vi "VI Server_Open VI Controls Refs_Labels_ApplicationRefInput.vi"(8 "error in (no error)":errorcluster, 10 "port number or service name (3363)":u16=3363, 11 "Target VI Path":path) -> (0 "error out":errorcluster, 3 "VI Server Cluster.OUT":T1)   [LabVIEW 2020, in "VI Server Toolkit LV2013.lvlib"]
doc: "Generates the VI Server Cluster with application input. Uses VI Server port to access application.\nThis VI used in compiled LabVIEW applications to access controls in LabVIEW development environment."
uses:
  VI Server Toolkit LV2013.lvlib
  VI Server_TypeDefs/VI Server_RefsCluster.ctl
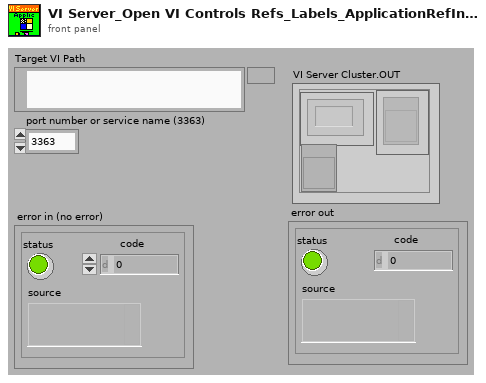
[diagram p1: front panel]
types:
  T1 = typedef "VI Server_RefsCluster.ctl" = cluster{"Labels":string[], "Refs":refnum<vi>[], "VI Ref":refnum<vi>}
  T2 = enum32{"invalid app kind", "Development System", "Run Time System", "Student Edition", "Embedded LabVIEW", "Evaluation", "Custom"}
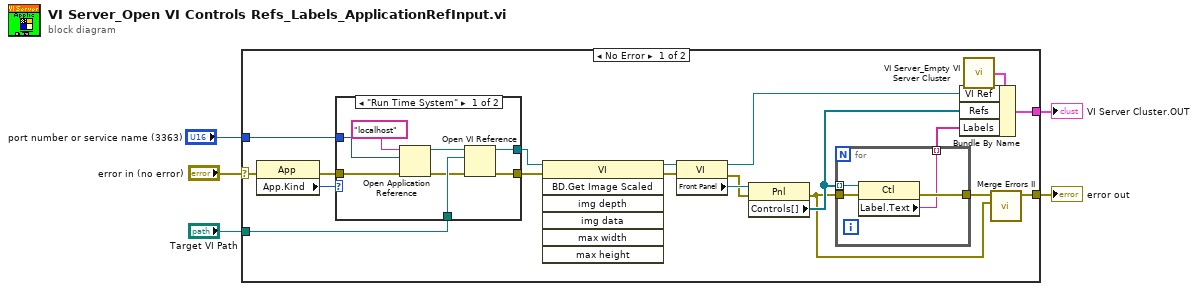
[diagram p0: block diagram]
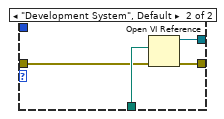
[diagram p2: hidden frame]
diagram:
  n1 = case shown="No Error" "error in (no error)" {
    selector: "error in (no error)" -> [w17 w41]
    tunnel: [w8 w41] -> w5
    tunnel: [w18 _] -> w4
    tunnel: "Target VI Path" -> [w19 _]
    tunnel: "port number or service name (3363)" -> [w11 _]
    frame No Error {
      n2 = property class="App"(error in=w17) -> (error out=w16:errorcluster, "App.Kind"=w7:T2)  [unwired: 1 in, 1 out]
      n3 = case shown="\"Run Time System\"" w7 {
        tunnel: [w32 w36] -> w14
        tunnel: [w31 w35] -> w15
        tunnel: w19 -> [w30 w34]
        tunnel: w16 -> [w26 w33]
        tunnel: w11 -> [w25 _]
        frame "Run Time System" {
          n4 = Open Application Reference(8:w26, 10:w25, 11:"localhost" ("machine name (\"\":  open local reference)")) -> (0:w29:errorcluster, 3:w28:refnum<vi>)  [unwired: 1 in]
          n5 = Open VI Reference(application reference (local)=w28, vi path=w30, error in (no error)=w29) -> (vi reference=w31:refnum<vi>, error out=w32:errorcluster)  [unwired: 3 out]
        }
        frame "Development System", Default {
          n6 = Open VI Reference(vi path=w34, error in (no error)=w33) -> (vi reference=w35:refnum<vi>, error out=w36:errorcluster)  [unwired: 4 out]
        }
      }
      n7 = invoke class="VI" method="BD.Get Image Scaled"(reference=w15, error in=w14) -> (reference out=w12:refnum<vi>, error out=w13:errorcluster)  [unwired: 5 in, 5 out]
      n8 = property class="VI"(reference=w12, error in=w13) -> (reference out=w21:refnum<vi>, error out=w23:errorcluster, "Front Panel"=w24:refnum<vi>)
      n9 = property class="Pnl"(reference=w24, error in=w23) -> (error out=w9:errorcluster, "Controls[]"=w20:refnum<vi>[])  [unwired: 1 out]
      n10 = for {
        tunnel: w20 -> [w40] mode=indexing
        tunnel: w9 -> [w39]
        tunnel: [w38] -> w10
        tunnel: [w37] -> w22 mode=indexing
        n11 = property class="Ctl"(reference=w40, error in=w39) -> (error out=w38:errorcluster, "Label.Text"=w37:string)  [unwired: 1 out]
      }
      n12 = call "VI Server_Empty VI Server Cluster.vi"() -> ("VI Server Cluster"=w6:T1)  [unwired: 7 in]
      n13 = Bundle By Name(cluster=w6, "VI Ref"=w21, "Refs"=w20, "Labels"=w22) -> (w18:T1)
      n14 = call "Merge Errors II.vi"("error in 2 (no error)"=w9, "error in 1 (no error)"=w10) -> ("error out.DUP"=w8:errorcluster)  [unwired: 4 in, 1 out]
    }
    frame Error {
    }
  }
  "error out" <- w5
  "VI Server Cluster.OUT" <- w4
